vi "pos_mm2unit.vi"(8 "error in (no error)":errorcluster, 10 "value in mm":dbl, 11 "Motor in":refnum<class "Motor.lvclass">) -> (0 "error out":errorcluster, 2 "value in unit":dbl, 3 "Motor out":refnum<class "Motor.lvclass">)   [LabVIEW 2016, in "Hardware.lvlib" / "Motor.lvlib" / "Motor.lvclass"]
uses:
  <userlib>/Common Components/Hardware/Motor/Motor/Motor.lvclass
  <userlib>/Common Components/Hardware/Motor/Motor/Motor.lvclass/Motor.ctl
  <userlib>/Common Components/Hardware/Motor/Motor/Accessor/Read display unit.vi
  <vilib>/Utility/error.llb/Error Cluster From Error Code.vi
  <vilib>/ErrorRing/Error Ring.xnode
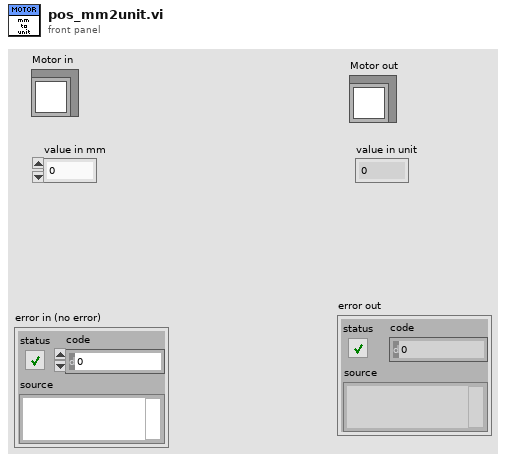
[diagram p1: front panel]
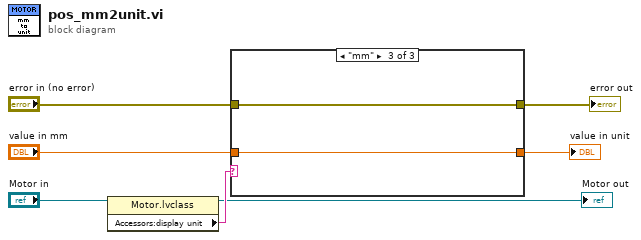
[diagram p0: block diagram]
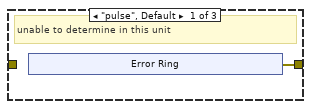
[diagram p2: hidden frame]
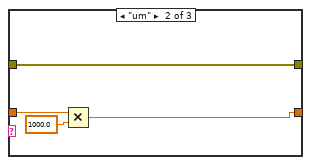
[diagram p3: hidden frame]
diagram:
  n1 = property class="Motor.lvclass"(reference="Motor in") -> (reference out=→"Motor out":refnum<class "Motor.lvclass">, "Accessors:display unit"=w4:string)  [unwired: 1 in, 1 out]
  n2 = case shown="\"mm\"" w4 {
    tunnel: "value in mm" -> [_ w16 w18]
    tunnel: [_ w14 w18] -> w6
    tunnel: "error in (no error)" -> [_ w13 w17]
    tunnel: [w8 w13 w17] -> w1
    frame "pulse", Default {
      # "unable to determine in this unit"
      n3 = xnode "Error Ring"() -> ("error out"=w8:errorcluster)
    }
    frame "um" {
      n4 = Multiply(x=w16, y=1000.0) -> (x*y=w14:dbl)
    }
    frame "mm" {
    }
  }
  "error out" <- w1
  "value in unit" <- w6
